vi "main.vi"() -> ()   [LabVIEW 2024]
uses:
  user_name.vi
panel:
  in  "Game Page":T1
  in  "New Game Difficulty Settings":T2 {"Difficulty" scale=1.0..10.0}
  in  "Choose How to Play":T3
  in  "Login Page":T4
  in  "Home Page":T5
  in  "stop":bool
  in  "Rules Page":cluster{"rules go back":bool}
  in  "Initial Page":T6
  # "TODO: Rules修改为vi独立弹出"
  # "TODO: 初始化时新建./data和./data/saves"
  # "Click to change avatar"
  # "Avatar Size: 72 * 72"
  # "进游戏以后难度会递增（闪烁间隔增加），此处决定初始难度"
  # "Score += Difficulty * 1 ?"
  # "Difficulty?"
  # "Your choice of difficulty will\nbe counted in the calculation\nof score"
  # "TODO: 是否给用户选项来选择\n是否使用云存档？默认云存档"
  # "How do you wanna start?"
  # "Your game will be\nautomatically saved\nto ./data/saves\nwhile playing"
  # "Login or Register"
  # "If you don't have an\naccount yet, we will\ncreate it for you"
  # "Simon Game"
  # "My highest score:"
  # "Achieved at:"
  # "Rules"
  # "1212123123123123123113\nSFdSAfsadfasdfasdfdsafasd\nafdasfsdafsdaf"
  # "Simon Game"
  # "Login to play"
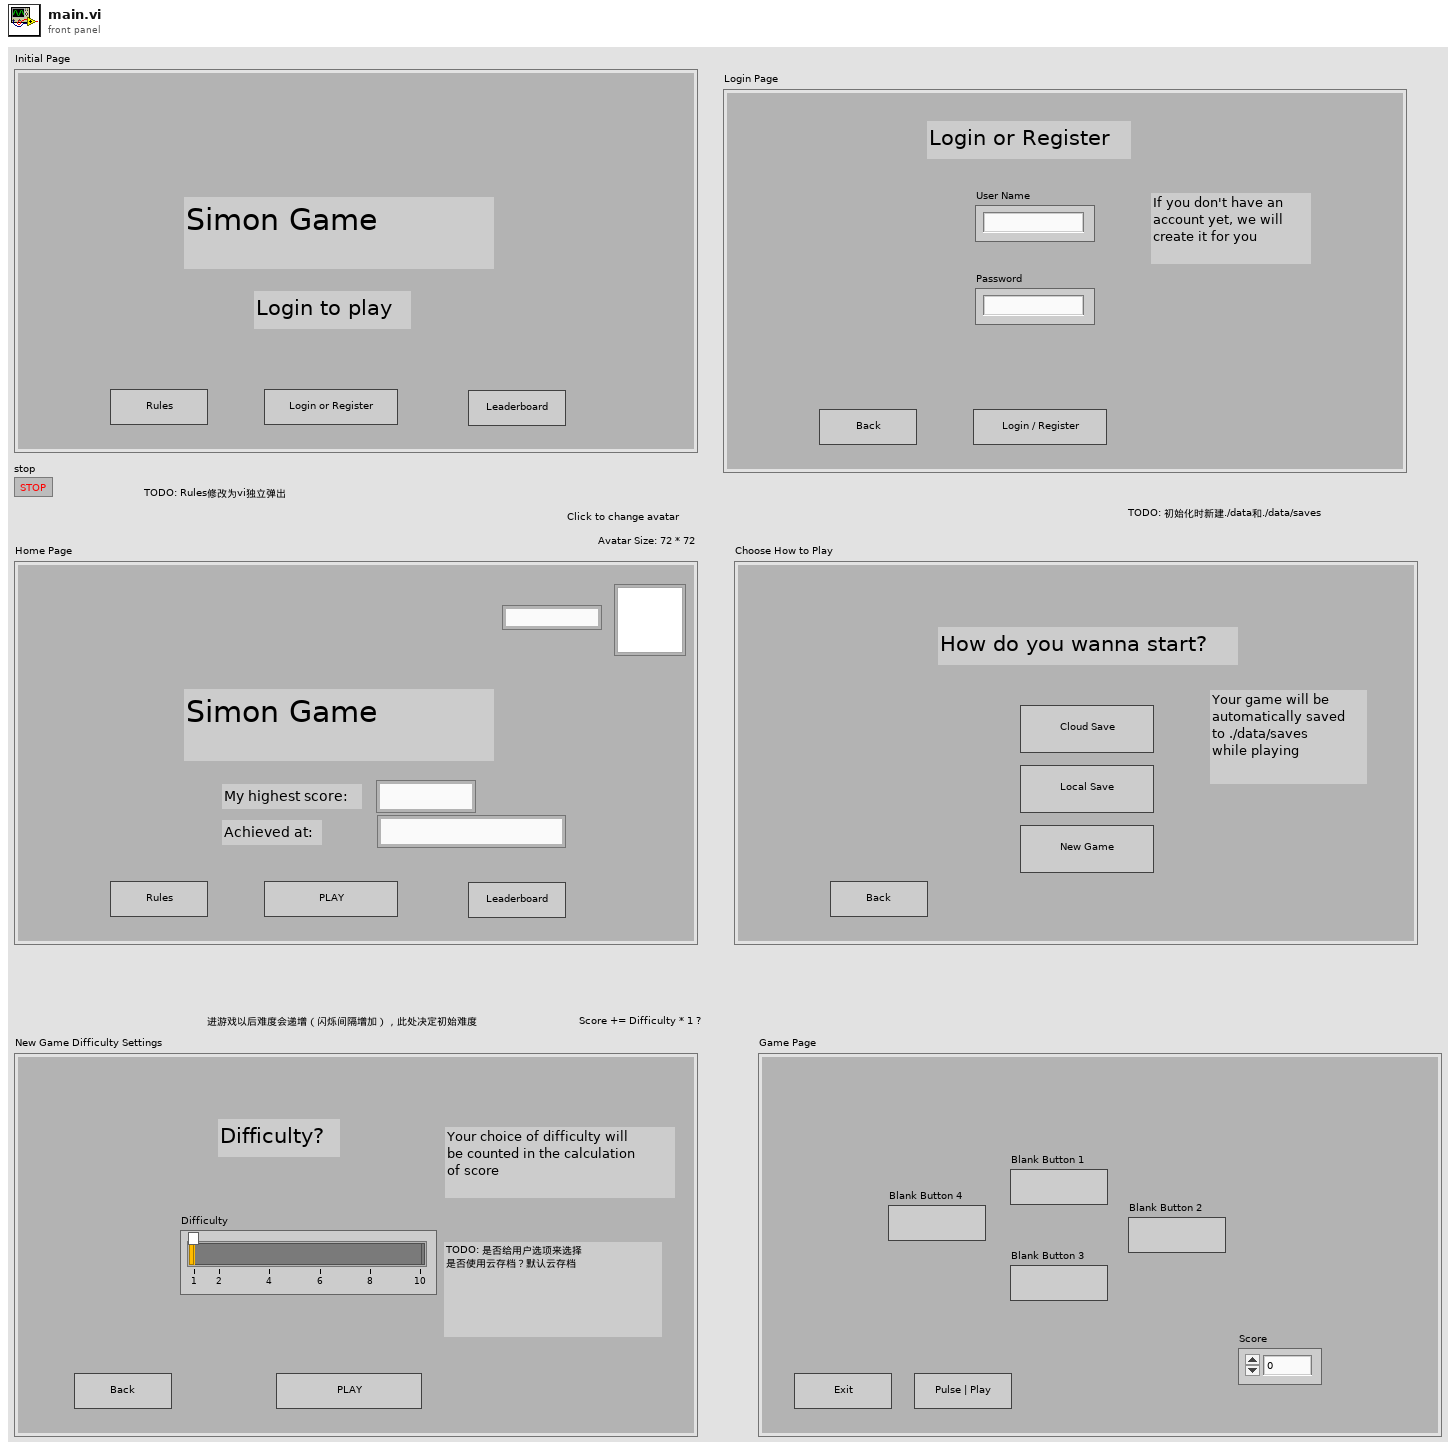
[diagram p1: front panel]
types:
  T1 = cluster{"Check Rules Button":bool, "Check Rules Button 2":bool, "Score":dbl, "Blank Button 1":bool, "Blank Button 2":bool, "Blank Button 3":bool, "Blank Button 4":bool}
  T2 = cluster{"Check Rules Button":bool, "Difficulty":dbl, "Check Rules Button 2":bool}
  T3 = cluster{"Check Rules Button":bool, "Cloud Save":bool, "Local Save":bool, "New Game":bool}
  T4 = cluster{"back to initial page":bool, "confirm login":bool, "User Name":string, "Password":string}
  T5 = cluster{"Check Rules Button":bool, "login button":bool, "Blank Button":bool, "User Name":string, "Avatar":picture, "user highest score":string, "user highest score achieved time":string}
  T6 = cluster{"Check Rules Button":bool, "login button":bool, "open leaderboard":bool}
  T7 = typedef "imagedata.ctl" = cluster{"image type":i32, "image depth":i32, "image":u8[], "mask":u8[], "colors":u32[], "Rectangle":cluster{"left":i16, "top":i16, "right":i16, "bottom":i16}}
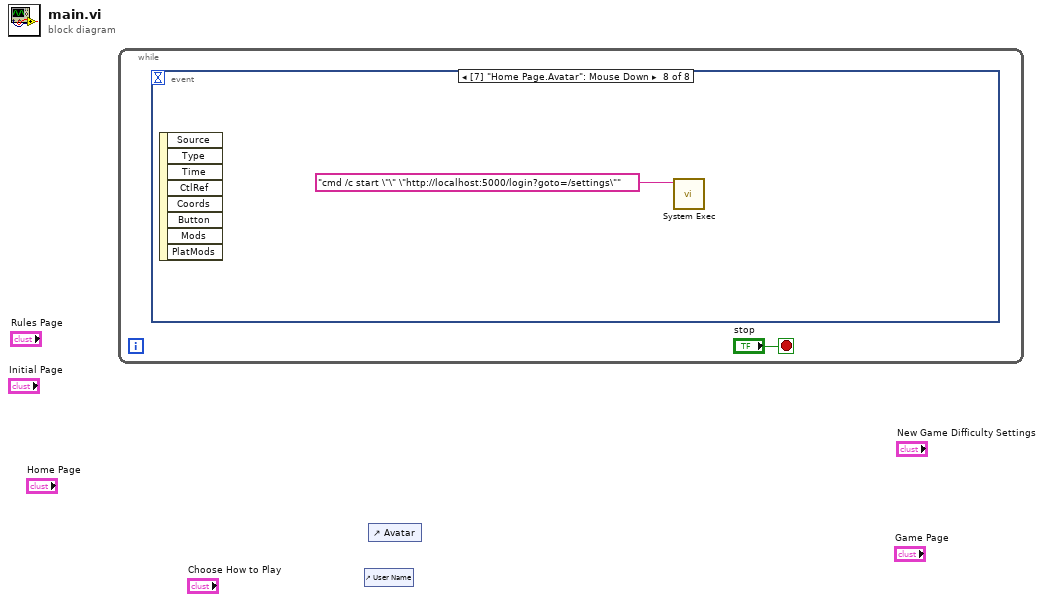
[diagram p0: block diagram]
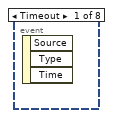
[diagram p2: hidden frame]
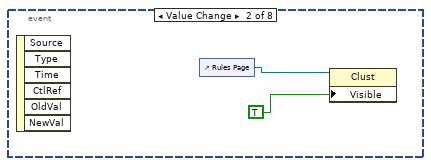
[diagram p3: hidden frame]
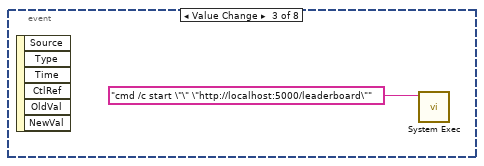
[diagram p4: hidden frame]
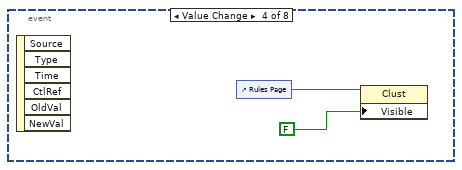
[diagram p5: hidden frame]
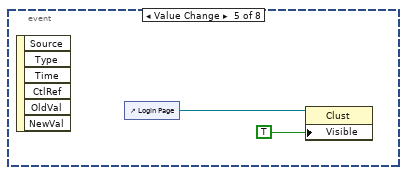
[diagram p6: hidden frame]
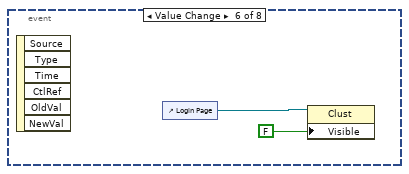
[diagram p7: hidden frame]
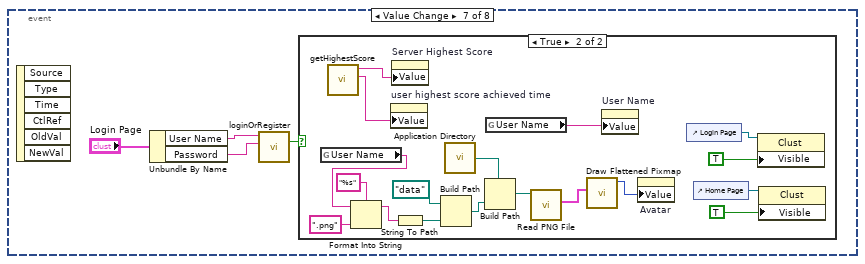
[diagram p8: hidden frame]
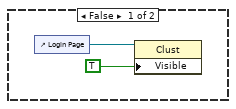
[diagram p9: hidden frame]
diagram:
  n1 = while {
    stop <- "stop" stop-if-true
    n2 = event shown="[7] \"Home Page.Avatar\": Mouse Down" {
      selector: _ -> [_ _ _ _ _ _ _ _]
      dyn-events: _ -> [_ _ _ _ _ _ _ _]
      timeout: _ -> [_ _ _ _ _ _ _ _]
      event Timeout {
        n3 = event-data() -> ()  [unwired: 1 in, 3 out]
      }
      event "Initial Page.Check Rules Button": Value Change {
        n4 = event-data() -> ()  [unwired: 1 in, 6 out]
        n5 = control-ref of="Rules Page"() -> (w3:refnum<vi>)
        n6 = property class="Clust"(reference=w3, "Visible"=TRUE) -> ()  [unwired: 1 in, 2 out]
      }
      event "Initial Page.open leaderboard": Value Change {
        n7 = event-data() -> ()  [unwired: 1 in, 6 out]
        n8 = call <vilib>:"System Exec.vi"("command line"="cmd /c start \"\" \"http://localhost:5000/leaderboard\"") -> ()  [unwired: 7 in, 4 out]
      }
      event "Rules Page.rules go back": Value Change {
        n9 = event-data() -> ()  [unwired: 1 in, 6 out]
        n10 = control-ref of="Rules Page"() -> (w5:refnum<vi>)
        n11 = property class="Clust"(reference=w5, "Visible"=FALSE) -> ()  [unwired: 1 in, 2 out]
      }
      event "Initial Page.login button": Value Change {
        n12 = event-data() -> ()  [unwired: 1 in, 6 out]
        n13 = control-ref of="Login Page"() -> (w7:refnum<vi>)
        n14 = property class="Clust"(reference=w7, "Visible"=TRUE) -> ()  [unwired: 1 in, 2 out]
      }
      event "Login Page.back to initial page": Value Change {
        n15 = event-data() -> ()  [unwired: 1 in, 6 out]
        n16 = control-ref of="Login Page"() -> (w9:refnum<vi>)
        n17 = property class="Clust"(reference=w9, "Visible"=FALSE) -> ()  [unwired: 1 in, 2 out]
      }
      event "Login Page.confirm login": Value Change {
        n18 = event-data() -> ()  [unwired: 1 in, 6 out]
        n19 = Unbundle By Name("Login Page") -> ("User Name"=w13:string, "Password"=w12:string)
        n20 = call "loginOrRegister.vi"("passwd"=w12, "uname"=w13) -> ("OK?"=w11:bool)  [unwired: 8 in, 1 out]
        n21 = case shown="True" w11 {
          frame False {
            n22 = control-ref of="Login Page"() -> (w15:refnum<vi>)
            n23 = property class="Clust"(reference=w15, "Visible"=TRUE) -> ()  [unwired: 1 in, 2 out]
          }
          frame True {
            n24 = global read "user_name.vi" "User Name"() -> (w21:string)
            n25 = call "getHighestScore.vi"() -> ("Highest Score Achineved Time"=w17:string, "Highest Score"=w34:string)  [unwired: 9 in, 1 out]
            n26 = Format Into String(format string="%s", initial string=w21, ".png" ("input 1")) -> (resulting string=w25:string)  [unwired: 1 in, 1 out]
            n27 = property on="user highest score achieved time" class="Str"("Value"=w17) -> ()  [unwired: 2 in, 2 out]
            n28 = property on="Server Highest Score" class="Str"("Value"=w34) -> ()  [unwired: 2 in, 2 out]
            n29 = String To Path(string=w25) -> (path=w27:path)
            n30 = Build Path(base path=path "data", name or relative path=w27) -> (appended path=w18:path)
            n31 = call <vilib>:"Application Directory.vi"() -> ("Application Directory"=w32:path)
            n32 = Build Path(base path=w32, name or relative path=w18) -> (appended path=w20:path)
            n33 = global read "user_name.vi" "User Name"() -> (w22:string)
            n34 = call <vilib>:"Read PNG File.vi"("path to PNG file"=w20) -> ("image data"=w19:T7)  [unwired: 8 in, 2 out]
            n35 = call <vilib>:"Draw Flattened Pixmap.vi"("image data"=w19) -> ("new picture"=w33:picture)  [unwired: 8 in]
            n36 = property on="User Name" class="Str"("Value"=w22) -> ()  [unwired: 2 in, 2 out]
            n37 = property on="Avatar" class="Pict"("Value"=w33) -> ()  [unwired: 2 in, 2 out]
            n38 = control-ref of="Login Page"() -> (w30:refnum<vi>)
            n39 = control-ref of="Home Page"() -> (w28:refnum<vi>)
            n40 = property class="Clust"(reference=w30, "Visible"=TRUE) -> ()  [unwired: 1 in, 2 out]
            n41 = property class="Clust"(reference=w28, "Visible"=TRUE) -> ()  [unwired: 1 in, 2 out]
          }
        }
      }
      event "Home Page.Avatar": Mouse Down {
        n42 = event-data() -> ()  [unwired: 1 in, 8 out]
        n43 = call <vilib>:"System Exec.vi"("command line"="cmd /c start \"\" \"http://localhost:5000/login?goto=/settings\"") -> ()  [unwired: 7 in, 4 out]
      }
    }
  }
  n44 = control-ref of="User Name"() -> ()  [unwired: 1 out]
  n45 = control-ref of="Avatar"() -> ()  [unwired: 1 out]
